vi "Run Action_Do.vi"(8 "error in (no error)":errorcluster, 10 "Project Builder in":refnum<class "Project Builder.lvclass">, 11 "Copy Build Product Action":refnum<class "Copy Build Product Action.lvclass">) -> (0 "error out":errorcluster, 1 "Success?":bool, 3 "Report":refnum<class "Report Data.lvclass">)   [LabVIEW 2020, in "ProjectBuilder.lvlib" / "Copy Build Product Action.lvclass"]
uses:
  Copy Build Product Action.lvclass
  Data/Report Data/Report Data.lvclass
  Project Builder/Project Builder.lvclass
  Build Named Build Specification/Build Named Build Specification Data/Build Named Build Specification Data.lvclass
  C:/Current projects/WS/LV32.2020..ProjectBuilder/Class/Data/Report Data/Report Data.lvclass
  Project Builder/Project Builder.lvclass/Project Builder.ctl
  Copy Build Product Action.lvclass/Copy Build Product Action.ctl
  Build Named Build Specification/Build Named Build Specification Data/Build Named Build Specification Data.lvclass/Build Named Build Specification Data.ctl
  PPL/HDH.ClassLoader.lvlibp
  ProjectBuilder.lvlib
  C:/Current projects/WS/LV32.2020..ProjectBuilder/Class/Build Named Build Specification/Build Named Build Specification Data/Build Named Build Specification Data.lvclass
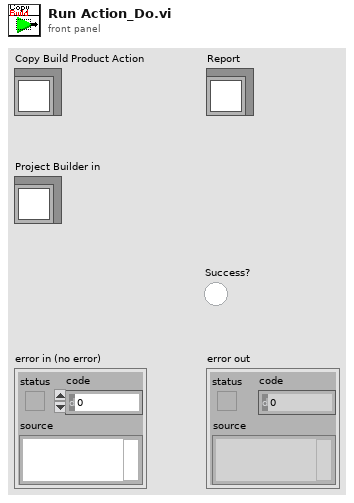
[diagram p1: front panel]
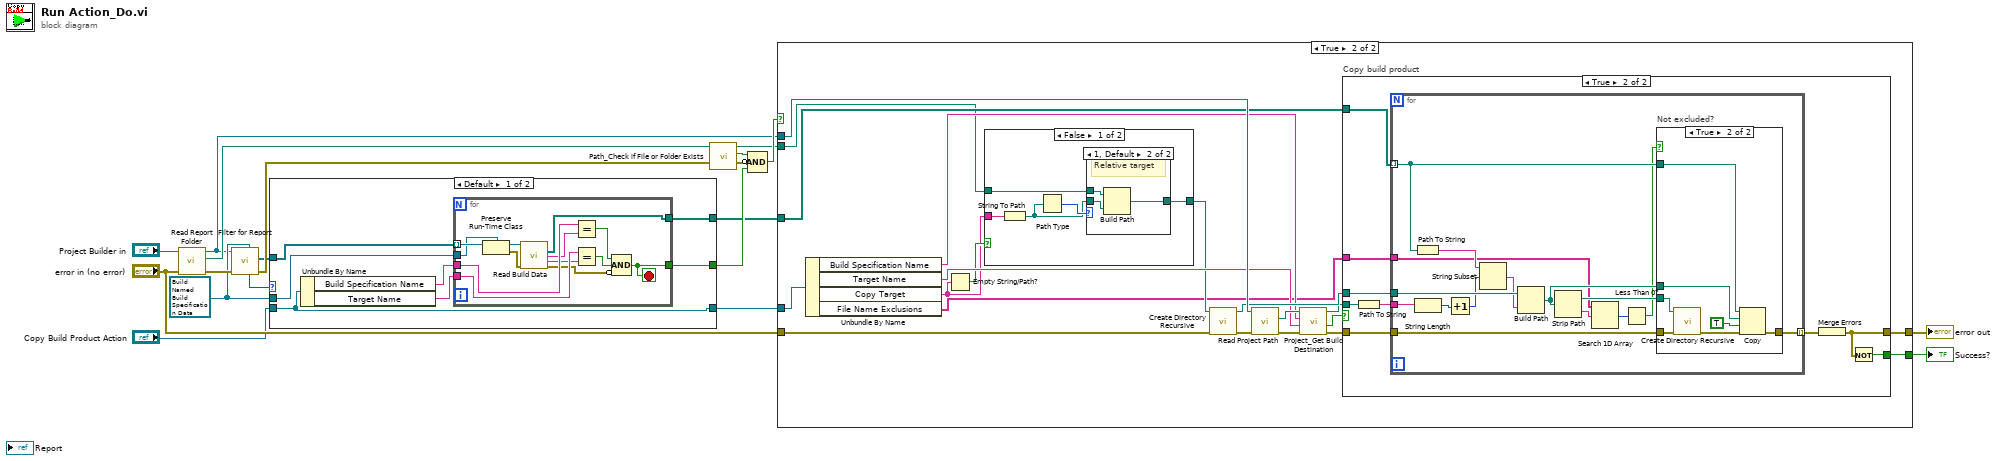
[diagram p0: block diagram]
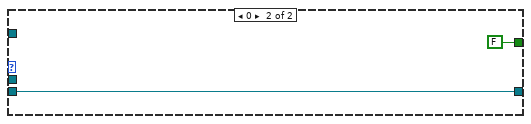
[diagram p2: hidden frame]
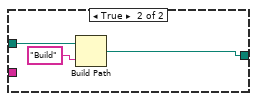
[diagram p5: hidden frame]
diagram:
  w6 = refnum<class "Build Named Build Specification Data.lvclass"> refnum ("ProjectBuilder.lvlib:Build Named Build Specification Data.lvclass")
  n1 = call "Read Report Folder.vi"("error in (no error)"="error in (no error)", "Project Builder in"="Project Builder in") -> ("error out"=w9:errorcluster, "Report Folder"=w16:path, "Project Builder out"=w2:refnum<class "Project Builder.lvclass">)  [unwired: 7 in]
  n2 = call "Filter for Report.vi"("Report Data Type (Report Data = Disable)"=w6, "error in (no error)"=w9, "Project Builder in"=w2) -> ("error out"=w8:errorcluster, "Filtered Reports"=w7:refnum<class "Report Data.lvclass">[], "Match Count"=w11:i32)  [unwired: 4 in, 2 out]
  n3 = case shown="Default" w11 {
    tunnel: [w20 FALSE] -> w10
    tunnel: w7 -> [w25 _]
    tunnel: w6 -> [w24 _]
    tunnel: "Copy Build Product Action" -> [w23 w39]
    tunnel: [w23 w39] -> w4
    tunnel: [w19 _] -> w3
    frame Default {
      n4 = Unbundle By Name(w23) -> ("Build Specification Name"=w22:string, "Target Name"=w21:string)
      n5 = for {
        tunnel: w25 -> [w38] mode=indexing
        tunnel: w24 -> [w37]
        tunnel: w22 -> [w34]
        tunnel: w21 -> [w32]
        tunnel: [w28] -> w19
        tunnel: [w26] -> w20
        stop <- w26 stop-if-true
        n6 = Preserve Run-Time Class(object in=w38, 2:w37) -> (object out=w36:refnum<class "Build Named Build Specification Data.lvclass">, error out=w35:errorcluster)  [unwired: 1 in]
        n7 = call "Read Build Data.vi"("Build Named Build Specification Data in"=w36, "error in (no error)"=w35) -> ("Generated files"=w28:path[], "Build Specification Name"=w33:string, "Target Name"=w31:string, "error out"=w27:errorcluster)  [unwired: 9 in, 1 out]
        n8 = Equal?(x=w34, y=w33) -> (x = y?=w30:bool)
        n9 = Equal?(x=w32, y=w31) -> (x = y?=w29:bool)
        n10 = Compound Arithmetic op=AND(w30, w29, invert w27) -> (w26:bool)
      }
    }
    frame 0 {
    }
  }
  n11 = call "Path_Check if File or Folder Exists.vi"("File or Folder Path in"=w16) -> ("File or Folder Found?"=w15:bool, "File or Folder Path dub"=w12:path)  [unwired: 9 in]
  n12 = Compound Arithmetic op=AND(w15, invert w8, w10) -> (w13:bool)
  n13 = case shown="True" w13 {
    tunnel: [w41 w55] -> w18
    tunnel: w4 -> [_ w61]
    tunnel: "error in (no error)" -> [w41 w57]
    tunnel: w12 -> [_ w45]
    tunnel: w3 -> [_ w59]
    tunnel: w2 -> [_ w60]
    tunnel: [_ w54] -> w1
    frame False {
    }
    frame True {
      n14 = Unbundle By Name(w61) -> ("Build Specification Name"=w49:string, "Target Name"=w48:string, "Copy Target"=w44:string, "File Name Exclusions"=w42:string[])
      n15 = Empty String/Path?(string/path=w44) -> (empty?=w46:bool)
      n16 = case shown="False" w46 {
        tunnel: w45 -> [w66 w72]
        tunnel: [w63 w71] -> w43
        tunnel: w44 -> [w62 _]
        frame False {
          n17 = String To Path(string=w62) -> (path=w64:path)
          n18 = Path Type(1:w64) -> (0:w65:i16)
          n19 = case shown="1, Default" w65 {
            tunnel: w64 -> [w67 w69]
            tunnel: w66 -> [_ w70]
            tunnel: [w67 w68] -> w63
            frame 0 {
              # "Absolute target"
            }
            frame 1, Default {
              # "Relative target"
              n20 = Build Path(base path=w70, name or relative path=w69) -> (appended path=w68:path)
            }
          }
        }
        frame True {
          n21 = Build Path(base path=w72, name or relative path="Build") -> (appended path=w71:path)
        }
      }
      n22 = call <vilib>:"Create Directory Recursive.vi"("error in (no error)"=w57, "directory"=w43) -> ("error out"=w56:errorcluster, "directory copy"=w58:path)  [unwired: 3 in, 1 out]
      n23 = call "Read Project Path.vi"("error in (no error)"=w56, "Project Builder in"=w60) -> ("error out"=w51:errorcluster, "Project Path"=w53:path)  [unwired: 7 in, 1 out]
      n24 = call "Project_Get Build Destination.vi"("error in(no error)"=w51, "Target Name(\"\"> My Computer)"=w48, "Build Specification Name"=w49, "Project Path"=w53) -> ("error out"=w50:errorcluster, "Success?"=w47:bool, "Build Destination"=w52:path)  [unwired: 5 in]
      n25 = case "Copy build product" shown="True" w47 {
        selector: w47 -> [w75 _]
        tunnel: w59 -> [_ w81]
        tunnel: w58 -> [_ w80]
        tunnel: [w74 w84] -> w55
        tunnel: [w75 w83] -> w54
        tunnel: w52 -> [_ w82]
        tunnel: w50 -> [w74 w78]
        tunnel: w42 -> [_ w76]
        frame False {
        }
        frame True {
          n26 = Path To String(path=w82) -> (string=w79:string)
          n27 = for {
            tunnel: w81 -> [w92] mode=indexing
            tunnel: w79 -> [w98]
            tunnel: w80 -> [w96]
            tunnel: w78 -> [w93]
            tunnel: [w90] -> w77 mode=indexing
            tunnel: w76 -> [w87]
            n28 = Path To String(path=w92) -> (string=w99:string)
            n29 = String Length(string=w98) -> (length=w97:i32)
            n30 = Increment(x=w97) -> (x+1=w89:i32)
            n31 = String Subset(string=w99, offset (0)=w89) -> (substring=w95:string)  [unwired: 1 in]
            n32 = Build Path(base path=w96, name or relative path=w95) -> (appended path=w91:path)
            n33 = Strip Path(path=w91) -> (stripped path=w94:path, name=w88:string)
            n34 = Search 1D Array(1D array=w87, element=w88) -> (index of element=w86:i32)  [unwired: 1 in]
            n35 = Less Than 0?(x=w86) -> (x < 0?=w85:bool)
            n36 = case "Not excluded?" shown="True" w85 {
              tunnel: w94 -> [_ w107]
              tunnel: w93 -> [w100 w106]
              tunnel: w92 -> [_ w104]
              tunnel: w91 -> [_ w103]
              tunnel: [w100 w101] -> w90
              frame False {
              }
              frame True {
                n37 = call <vilib>:"Create Directory Recursive.vi"("error in (no error)"=w106, "directory"=w107) -> ("error out"=w102:errorcluster)  [unwired: 3 in, 2 out]
                n38 = Copy(8:w102, 9:TRUE ("overwrite (F)"), 10:w103, 11:w104) -> (0:w101:errorcluster)  [unwired: 1 in, 2 out]
              }
            }
          }
          n39 = Merge Errors(w77) -> (w84:errorcluster)
          n40 = Not(x=w84) -> (.not. x?=w83:bool)
        }
      }
    }
  }
  "error out" <- w18
  "Success?" <- w1
